vi "tarea_1_ft.vi"() -> ()   [LabVIEW 2019]
uses:
  <vilib>/Analysis/baseanly.llb/A x Vector.vi
  <vilib>/Analysis/baseanly.llb/Real Dot Product.vi
  <vilib>/Analysis/NI_AALBase.lvlib
panel:
  out "SIMULACIÓN SISTEMA DINÁMICO":cluster{"u(t)":dbl, "y":dbl}(graph)
  out "y(t)":dbl format="%.2f"
  in  "u(t)":dbl
  in  "Den":dbl[](array[numeric])
  in  "Num":dbl[](array[numeric])
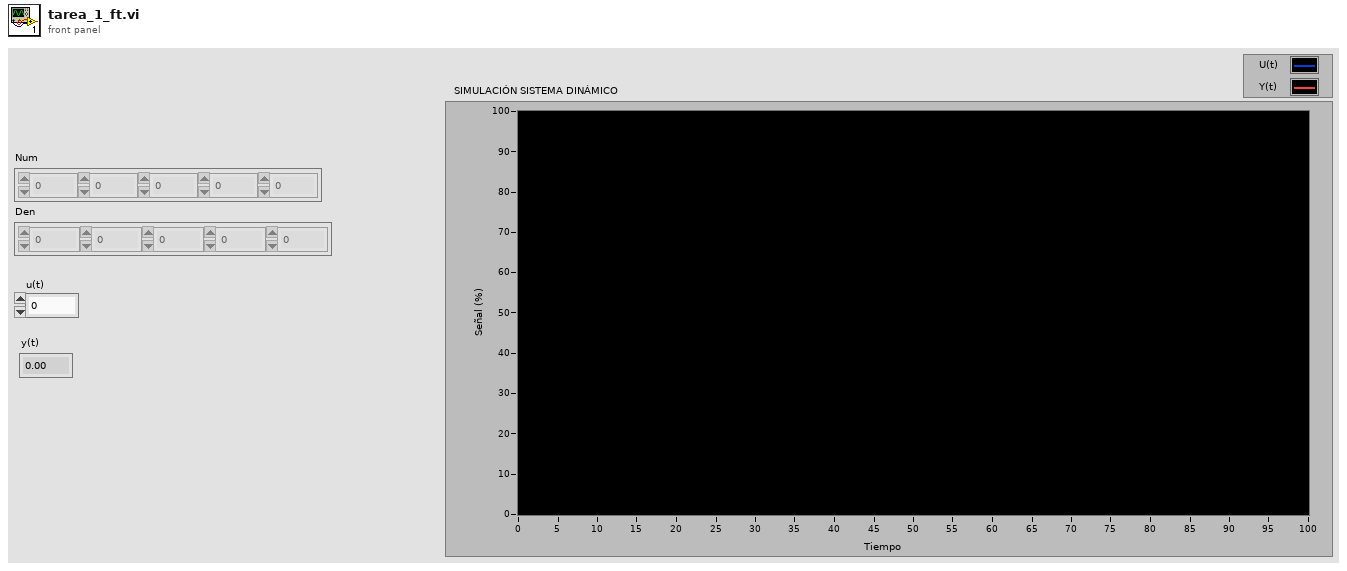
[diagram p1: front panel]
types:
  T1 = typedef "NI_Matrix.lvlib/RealMatrix.ctl" = dbl[][]
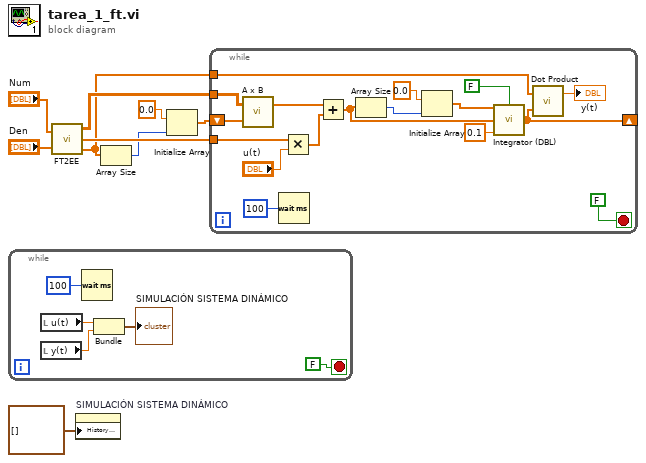
[diagram p0: block diagram]
diagram:
  n1 = while {
    stop <- FALSE stop-if-true
    n2 = local read "u(t)"() -> (w14:dbl)
    n3 = local read "y(t)"() -> (w13:dbl)
    n4 = Wait (ms)(milliseconds to wait=u32 100) -> ()  [unwired: 1 out]
    n5 = Bundle("u(t)"=w14, "y(t)"=w13) -> (→"SIMULACIÓN SISTEMA DINÁMICO":cluster{"u(t)":dbl, "y(t)":dbl})  [unwired: 1 in]
  }
  n6 = call "FT2EE.vi"("NUMERADOR"="Num", "DENOMINADOR"="Den") -> ("A"=w7:T1, "B"=w6:dbl[], "C"=w4:dbl[])
  n7 = property on="SIMULACIÓN SISTEMA DINÁMICO" class="WFChart (strict)"("History Data"=cluster{"u(t)":dbl, "y":dbl}[] []) -> ()  [unwired: 2 in, 2 out]
  n8 = Array Size(array=w4) -> (size(s)=w2:i32)
  n9 = Initialize Array(0.0 ("element"), w2) -> (w1:dbl[])
  n10 = while {
    shift-right: [w16] -> _
    shift-left: w1 -> [w18]
    tunnel: w7 -> [w30]
    tunnel: w6 -> [w28]
    tunnel: w4 -> [w25]
    stop <- FALSE stop-if-true
    n11 = call-poly <vilib>:"A x B.vi"("Vector"=w18, "A"=w30) -> ("A x Vector"=w17:dbl[])  [unwired: 1 out]
    n12 = Wait (ms)(milliseconds to wait=u32 100) -> ()  [unwired: 1 out]
    n13 = Multiply(x=w28, y="u(t)") -> (x*y=w27:dbl[])
    n14 = Add(x=w17, y=w27) -> (x+y=w22:dbl[])
    n15 = Array Size(array=w22) -> (size(s)=w21:i32)
    n16 = Initialize Array(0.0 ("element"), w21) -> (w19:dbl[])
    n17 = call "Integrator (DBL).vi"("initial condition"=w19, "initialize"=FALSE, "input point"=w22, "dt"=0.1) -> ("output"=w16:dbl[])  [unwired: 11 in]
    n18 = call-poly <vilib>:"Dot Product.vi"("Y Vector"=w16, "X Vector"=w25) -> ("X * Y"=→"y(t)":dbl)  [unwired: 1 out]
  }
